vi "Get Clump Precursors.vi"(8 "error in (no error)":errorcluster, 11 "Outputs.Channel Data.Coils":T4[](array[typedef])) -> (0 "error out":errorcluster, 3 "Clump Precursors":T1[](array[typedef]))   [LabVIEW 2015]
uses:
  Shared/Controls/Data Model/Channel.ctl
  System Explorer/SubVIs/Modbus Type.ctl
  <vilib>/NI Veristand/Custom Device API/Custom Device Channel Type.ctl
  Shared/Controls/Data Model/Mapping.ctl
  Shared/Controls/Data Model/DataType.ctl
  <vilib>/NI Veristand/Custom Device API/Custom Device Item Ref.ctl
  Clump Precursor.ctl
  Shared/Modbus Master Shared.lvlib
  <vilib>/NI VeriStand/Custom Device API/Custom Device API.lvlib
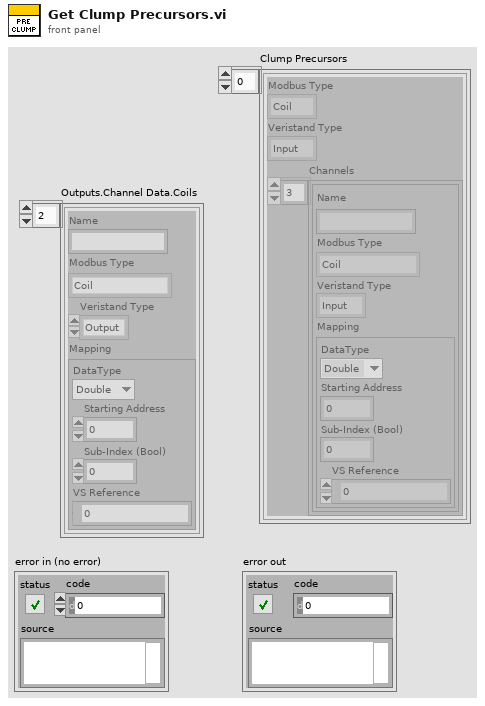
[diagram p1: front panel]
types:
  T1 = typedef "Modbus Master Shared.lvlib/Clump Precursor.ctl" = cluster{"Modbus Type":T2, "Veristand Type":T3, "Channels":T4[]}
  T2 = typedef "Modbus Master Shared.lvlib/Modbus Type.ctl" = enum16{"Coil", "Discrete Input", "Holding Register", "Input Register"}
  T3 = typedef "Custom Device API.lvlib/Custom Device Channel Type.ctl" = enum16{"Input", "Output"}
  T4 = typedef "Modbus Master Shared.lvlib/Channel.ctl" = cluster{"Name":string, "Modbus Type":T2, "Veristand Type":T3, "Mapping":T5}
  T5 = typedef "Modbus Master Shared.lvlib/Mapping.ctl" = cluster{"DataType":T6, "Starting Address":u16, "Sub-Index (Bool)":u16, "VS Reference":T7}
  T6 = typedef "Modbus Master Shared.lvlib/DataType.ctl" = enum16{"Double", "Single", "I64", "I32", "I16", "I8", "U64", "U32", "U16", "U8", "Boolean"}
  T7 = typedef "Custom Device API.lvlib/Custom Device Item Ref.ctl" = u64
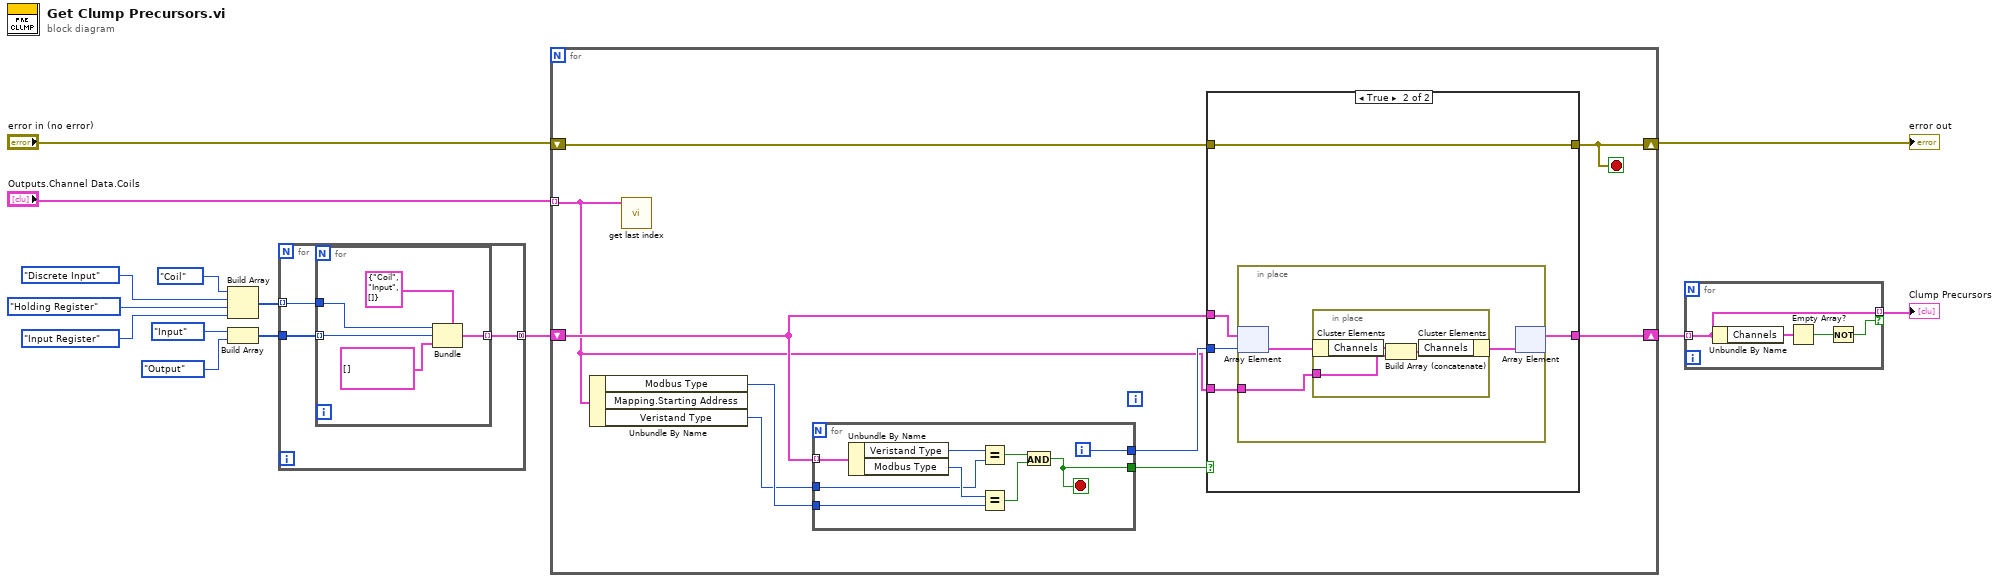
[diagram p0: block diagram]
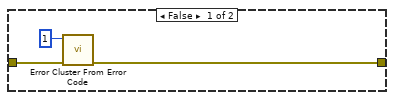
[diagram p2: hidden frame]
diagram:
  n1 = Build Array(Modbus_Type."Coil" ("Modbus Type"), Modbus_Type."Discrete Input" ("Modbus Type"), Modbus_Type."Holding Register" ("Modbus Type"), Modbus_Type."Input Register" ("Modbus Type")) -> (w4:T2[])
  n2 = Build Array(Custom_Device_Channel_Type."Input" ("Veristand Type"), Custom_Device_Channel_Type."Output" ("element")) -> (w3:T3[])
  n3 = for {
    tunnel: w4 -> [w17] mode=indexing
    tunnel: w3 -> [w16]
    tunnel: [w15] -> w2 mode=concatenating
    n4 = for {
      tunnel: w17 -> [w22]
      tunnel: w16 -> [w21] mode=indexing
      tunnel: [w20] -> w15 mode=indexing
      n5 = Bundle(cluster=T1 {"Modbus Type"=enum."Coil", "Veristand Type"=enum."Input", "Channels"=[]} ("output cluster"), "Modbus Type"=w22, "Veristand Type"=w21, "Channels"=T4[] [] ("Outputs.Channel Data.Coils")) -> (w20:T1)
    }
  }
  n6 = for {
    tunnel: "Outputs.Channel Data.Coils" -> [w23] mode=indexing
    shift-right: [w28] -> w5
    shift-left: w2 -> [w29]
    shift-right: [w27] -> w6
    shift-left: "error in (no error)" -> [w31]
    stop <- w27 stop-if-true
    n7 = Unbundle By Name(w23) -> ("Modbus Type"=w25:T2, "Veristand Type"=w24:T3)  [unwired: 1 out]
    n8 = call "get last index.vi"("Channel"=w23) -> ()  [unwired: 10 in, 1 out]
    n9 = for {
      tunnel: w29 -> [w54] mode=indexing
      tunnel: w25 -> [w51]
      tunnel: [w48] -> w26
      tunnel: [w47] -> w30
      tunnel: w24 -> [w46]
      i -> [w48]
      stop <- w47 stop-if-true
      n10 = Unbundle By Name(w54) -> ("Veristand Type"=w52:T3, "Modbus Type"=w53:T2)
      n11 = Equal?(x=w52, y=w46) -> (x = y?=w49:bool)
      n12 = Equal?(x=w53, y=w51) -> (x = y?=w50:bool)
      n13 = And(x=w49, y=w50) -> (x .and. y?=w47:bool)
    }
    n14 = case shown="True" w30 {
      tunnel: w29 -> [_ w38]
      tunnel: [_ w37] -> w28
      tunnel: [w34 w39] -> w27
      tunnel: w31 -> [w33 w39]
      tunnel: w26 -> [_ w36]
      tunnel: w23 -> [_ w35]
      frame False {
        n15 = call <vilib>:"Error Cluster From Error Code.vi"("error in (no error)"=w33, "error code (0)"=1) -> ("error out"=w34:errorcluster)  [unwired: 7 in]
      }
      frame True {
        n16 = in-place {
          in-place-border: w35 -> [w40]
          n17 = in-place-array #1(w38, w36) -> (w42:T1)
          n18 = in-place {
            in-place-border: w40 -> [w43]
            n19 = in-place-cluster #2(w42) -> ("Channels"=w45:T4[])
            n20 = Build Array (concatenate)(w45, w43) -> (w44:T4[])
            n21 = in-place-cluster #2("Channels"=w44) -> (w41:T1)
          }
          n22 = in-place-array #1(w41) -> (w37:T1[])  [unwired: 1 out]
        }
      }
    }
  }
  "error out" <- w6
  n23 = for {
    tunnel: [w58] -> w14 mode=indexing if=w56
    tunnel: w5 -> [w58] mode=indexing
    n24 = Unbundle By Name(w58) -> ("Channels"=w57:T4[])
    n25 = Empty Array?(array=w57) -> (empty?=w55:bool)
    n26 = Not(x=w55) -> (.not. x?=w56:bool)
  }
  "Clump Precursors" <- w14
